vi "determine required data sets.vi"(8 "error in":errorcluster, 10 "Slave Info List":T2(array[cluster]), 11 "channels":refnum<class "Profibus channel.lvclass">[](array[class])) -> (0 "error out":errorcluster, 3 "slave data subsets":T1[](array[typedef]))   [LabVIEW 2013, in "Profibus Module runtime.lvclass"]
uses:
  Profibus Module runtime.lvclass
  channel/Profibus channel.lvclass
  required data sets.ctl
  channel/Profibus channel.lvclass/Profibus channel.ctl
  <vilib>/NI/Tag Bus/tag/tag descriptor.lvclass/tag descriptor.ctl
  <vilib>/NI/Tag Bus Module Framework/channel/TBM channel.lvclass/TBM channel.ctl
  channel/Read byte.vi
  <vilib>/NI/Tag Bus/tag/read data type.vi
  <vilib>/NI/Tag Bus Module Framework/channel/Read channel classification.vi
  channel/Read slave.vi
  <vilib>/NI/Tag Bus/tag/read tag name.vi
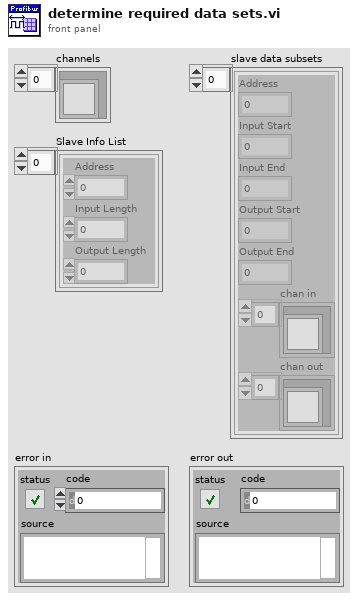
[diagram p1: front panel]
types:
  T1 = typedef "Profibus Module runtime.lvclass/required data sets.ctl" = cluster{"Address":i8, "Input Start":u8, "Input End":u8, "Output Start":u8, "Output End":u8, "chan in":refnum<class "Profibus channel.lvclass">[], "chan out":refnum<class "Profibus channel.lvclass">[]}
  T2 = cluster{"Address":i8, "Input Length":u8, "Output Length":u8}[]
  T3 = typedef "tag bus.lvlib/tag descriptor.lvclass/Data Type.ctl" = enum16{"Double", "Single", "I64", "I32", "I16", "I8", "U64", "U32", "U16", "U8", "Boolean", "String", "Array of Double", "Array of Single", "Array of I64", "Array of I32", "Array of I16", "Array of I8", "Array of U64", "Array of U32", "Array of U16", "Array of U8", "Array of Boolean", "Array of String"}
  T4 = typedef "TBM channel.lvclass/channel classification.ctl" = enum16{"input data", "output data", "processing parameter", "processing result"}
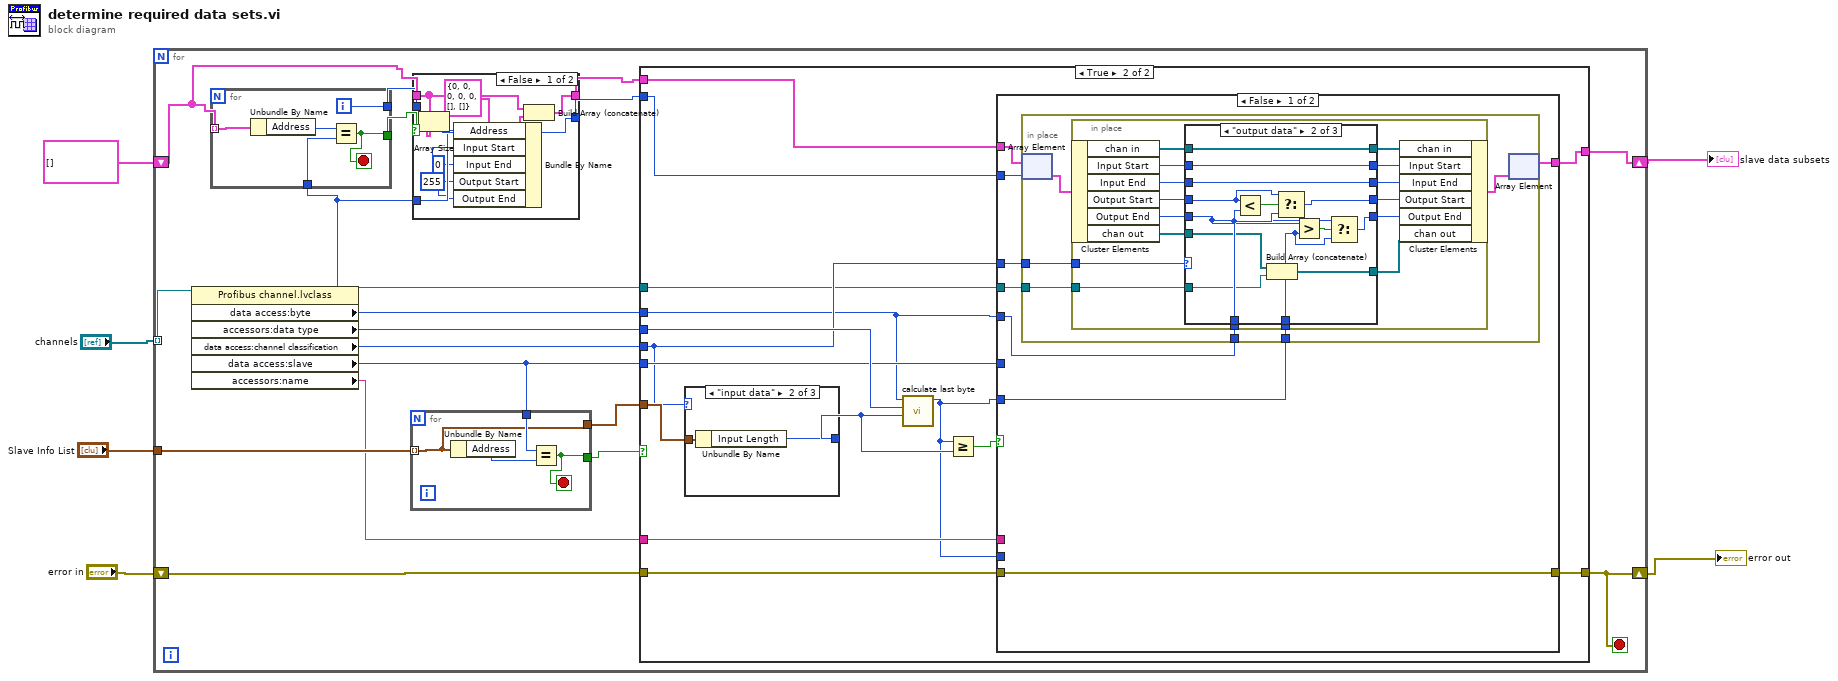
[diagram p0: block diagram]
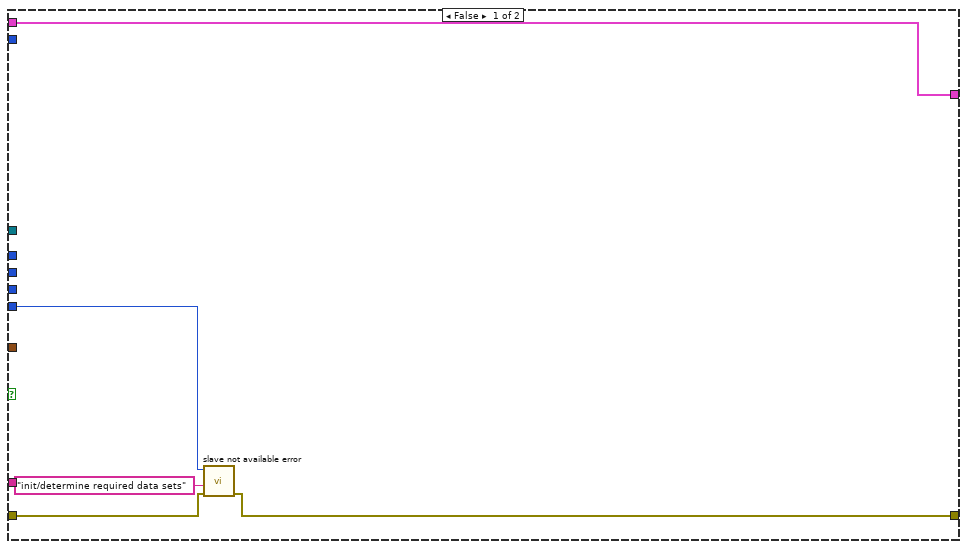
[diagram p3: hidden frame]
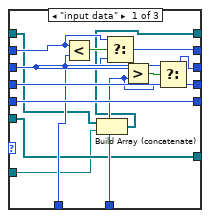
[diagram p4: hidden frame]
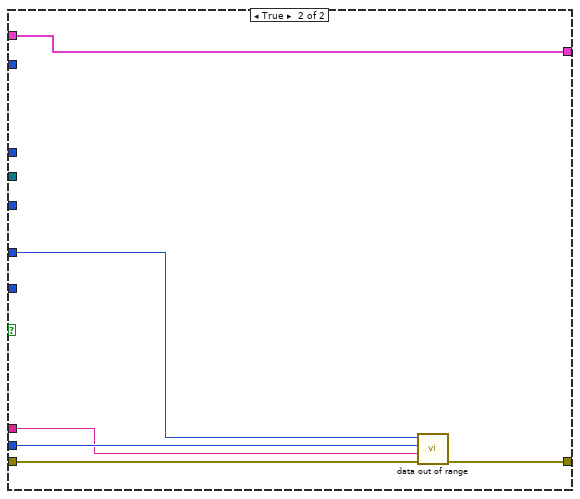
[diagram p6: hidden frame]
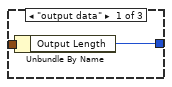
[diagram p7: hidden frame]
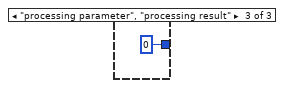
[diagram p8: hidden frame]
diagram:
  n1 = for {
    tunnel: "Slave Info List" -> [w24]
    tunnel: "channels" -> [w23] mode=indexing
    shift-right: [w21] -> w3
    shift-left: "error in" -> [w22]
    shift-right: [w9] -> w1
    shift-left: T1[] [] -> [w13]
    stop <- w21 stop-if-true
    n2 = property class="Profibus channel.lvclass"(reference=w23) -> (reference out=w7:refnum<class "Profibus channel.lvclass">, "data access:byte"=w16:i32, "accessors:data type"=w17:T3, "data access:channel classification"=w18:T4, "data access:slave"=w10:i8, "accessors:name"=w8:string)  [unwired: 1 in, 1 out]
    n3 = for {
      tunnel: w13 -> [w37] mode=indexing
      tunnel: w10 -> [w38]
      tunnel: [w36] -> w15
      tunnel: [w35] -> w11
      i -> [w35]
      stop <- w36 stop-if-true
      n4 = Unbundle By Name(w37) -> ("Address"=w39:i8)
      n5 = Equal?(x=w39, y=w38) -> (x = y?=w36:bool)
    }
    n6 = for {
      tunnel: w24 -> [w136] mode=indexing
      tunnel: w10 -> [w137]
      tunnel: [w136] -> w19
      tunnel: [w135] -> w20
      stop <- w135 stop-if-true
      n7 = Unbundle By Name(w136) -> ("Address"=w138:i8)
      n8 = Equal?(x=w137, y=w138) -> (x = y?=w135:bool)
    }
    n9 = case shown="False" w15 {
      tunnel: [w32 w34] -> w14
      tunnel: w13 -> [w31 w34]
      tunnel: [w30 w33] -> w12
      tunnel: w11 -> [_ w33]
      tunnel: w10 -> [w27 _]
      frame False {
        w25 = u8 255 ("Output Start")
        w26 = u8 0 ("Input End")
        n10 = Array Size(array=w31) -> (size(s)=w30:i32)
        n11 = Bundle By Name(cluster=T1 {"Address"=0, "Input Start"=0, "Input End"=0, "Output Start"=0, "Output End"=0, "chan in"=[], "chan out"=[]} ("Slave Info"), "Address"=w27, "Input Start"=w25, "Input End"=w26, "Output Start"=w25, "Output End"=w26) -> (w28:T1)
        n12 = Build Array (concatenate)(w31, w28) -> (w32:T1[])
      }
      frame True {
      }
    }
    n13 = case shown="True" w20 {
      tunnel: w22 -> [w44 w55]
      tunnel: [w42 w52] -> w21
      tunnel: w10 -> [w41 w51]
      tunnel: w19 -> [_ w59]
      tunnel: w18 -> [_ w48]
      tunnel: w17 -> [_ w58]
      tunnel: w16 -> [_ w47]
      tunnel: w14 -> [w40 w53]
      tunnel: w12 -> [_ w49]
      tunnel: [w40 w54] -> w9
      tunnel: w8 -> [_ w50]
      tunnel: w7 -> [_ w45]
      frame False {
        n14 = call "slave not available error.vi"("error in"=w44, "source"="init/determine required data sets", "slave"=w41) -> ("error out"=w42:errorcluster)  [unwired: 8 in]
      }
      frame True {
        n15 = case shown="\"input data\"" w48 {
          tunnel: w59 -> [w131 w133 _]
          tunnel: [w130 w132 u8 0 ("Output Length")] -> w57
          frame "output data" {
            n16 = Unbundle By Name(w131) -> ("Output Length"=w130:u8)
          }
          frame "input data" {
            n17 = Unbundle By Name(w133) -> ("Input Length"=w132:u8)
          }
          frame "processing parameter", "processing result" {
          }
        }
        n18 = call "calculate last byte.vi"("buffer length"=w57, "type"=w58, "byte in"=w47) -> ("last byte"=w46:i32)  [unwired: 8 in]
        n19 = Greater Or Equal?(x=w46, y=w57) -> (x >= y?=w56:bool)
        n20 = case shown="False" w56 {
          tunnel: w55 -> [w61 w129]
          tunnel: [w66 w128] -> w54
          tunnel: w53 -> [w67 w128]
          tunnel: [w61 w127] -> w52
          tunnel: w51 -> [_ w126]
          tunnel: w46 -> [_ w125]
          tunnel: w50 -> [_ w124]
          tunnel: w49 -> [w65 _]
          tunnel: w48 -> [w64 _]
          tunnel: w47 -> [w63 _]
          tunnel: w46 -> [w62 _]
          tunnel: w45 -> [w60 _]
          frame False {
            n21 = in-place {
              in-place-border: w64 -> [w71]
              in-place-border: w63 -> [w70]
              in-place-border: w62 -> [w69]
              in-place-border: w60 -> [w68]
              n22 = in-place-array #1(w67, w65) -> (w73:T1)
              n23 = in-place {
                in-place-border: w71 -> [w89]
                in-place-border: w70 -> [w80]
                in-place-border: w69 -> [w79]
                in-place-border: w68 -> [w75]
                n24 = in-place-cluster #2(w73) -> ("chan in"=w77:refnum<class "Profibus channel.lvclass">[], "Input Start"=w88:u8, "Input End"=w85:u8, "Output Start"=w84:u8, "Output End"=w81:u8, "chan out"=w76:refnum<class "Profibus channel.lvclass">[])
                n25 = case shown="\"output data\"" w89 {
                  tunnel: w88 -> [w99 w117 w123]
                  tunnel: [w96 w117 w123] -> w87
                  tunnel: [w97 w116 w122] -> w86
                  tunnel: w85 -> [w98 w116 w122]
                  tunnel: w84 -> [w103 w114 w121]
                  tunnel: [w103 w112 w121] -> w83
                  tunnel: [w102 w108 w120] -> w82
                  tunnel: w81 -> [w102 w110 w120]
                  tunnel: w80 -> [w94 w113 _]
                  tunnel: w79 -> [w95 w109 _]
                  tunnel: [w90 w107 w118] -> w78
                  tunnel: w77 -> [w91 w107 w118]
                  tunnel: w76 -> [w93 w106 w119]
                  tunnel: w75 -> [w92 w105 _]
                  tunnel: [w93 w104 w119] -> w74
                  frame "input data" {
                    n26 = Less?(x=w99, y=w94) -> (x < y?=w101:bool)
                    n27 = Build Array (concatenate)(w91, w92) -> (w90:refnum<class "Profibus channel.lvclass">[])
                    n28 = Select(t=w99, s=w101, f=w94) -> (s? t:f=w96:i32)
                    n29 = Greater?(x=w98, y=w95) -> (0:w100:bool)
                    n30 = Select(t=w98, s=w100, f=w95) -> (s? t:f=w97:i32)
                  }
                  frame "output data" {
                    n31 = Less?(x=w114, y=w113) -> (x < y?=w115:bool)
                    n32 = Build Array (concatenate)(w106, w105) -> (w104:refnum<class "Profibus channel.lvclass">[])
                    n33 = Select(t=w114, s=w115, f=w113) -> (s? t:f=w112:i32)
                    n34 = Greater?(x=w110, y=w109) -> (0:w111:bool)
                    n35 = Select(t=w110, s=w111, f=w109) -> (s? t:f=w108:i32)
                  }
                  frame Default {
                  }
                }
                n36 = in-place-cluster #2("chan in"=w78, "Input Start"=w87, "Input End"=w86, "Output Start"=w83, "Output End"=w82, "chan out"=w74) -> (w72:T1)
              }
              n37 = in-place-array #1(w72) -> (w66:T1[])  [unwired: 1 out]
            }
          }
          frame True {
            n38 = call "data out of range.vi"("error in"=w129, "source"=w124, "byte"=w125, "slave"=w126) -> ("error out"=w127:errorcluster)  [unwired: 7 in]
          }
        }
      }
    }
  }
  "error out" <- w3
  "slave data subsets" <- w1
